vi "Start LabVIEW.vi"(8 "Error In":errorcluster, 11 "Install LV Data":T1={"SSH Session"=refnum, "Status Log"="", "Detailed Log"="", "Credentials"={"Hostname or IP"="192.168.7.2", "Username"="root", "Password"=""}, "Target Info"={"OS Version"="", "CPU"="", "Systemd Version"="", "Internet Access"=FALSE, "Device Type"="", "LV Installed Ver"="", "LV Available Ver"="", "LV Upgrade Available"=FALSE, "Hostname"="", "NIC Info"=[]}, "Reboot Required?"=FALSE}) -> (0 "Error Out":errorcluster, 1 "Log":string, 2 "LV Running?":bool, 3 "Install LV Data":T1={"SSH Session"=refnum, "Status Log"="", "Detailed Log"="", "Credentials"={"Hostname or IP"="192.168.7.2", "Username"="root", "Password"=""}, "Target Info"={"OS Version"="", "CPU"="", "Systemd Version"="", "Internet Access"=FALSE, "Device Type"="", "LV Installed Ver"="", "LV Available Ver"="", "LV Upgrade Available"=FALSE, "Hostname"="", "NIC Info"=[]}, "Reboot Required?"=FALSE})   [LabVIEW 2020, in "LMH-LINX.lvlib"]
uses:
  LMH-LINX.lvlib
  Install LV Data.ctl
  Target Info.ctl
  NIC Info.ctl
  NIC Mode.ctl
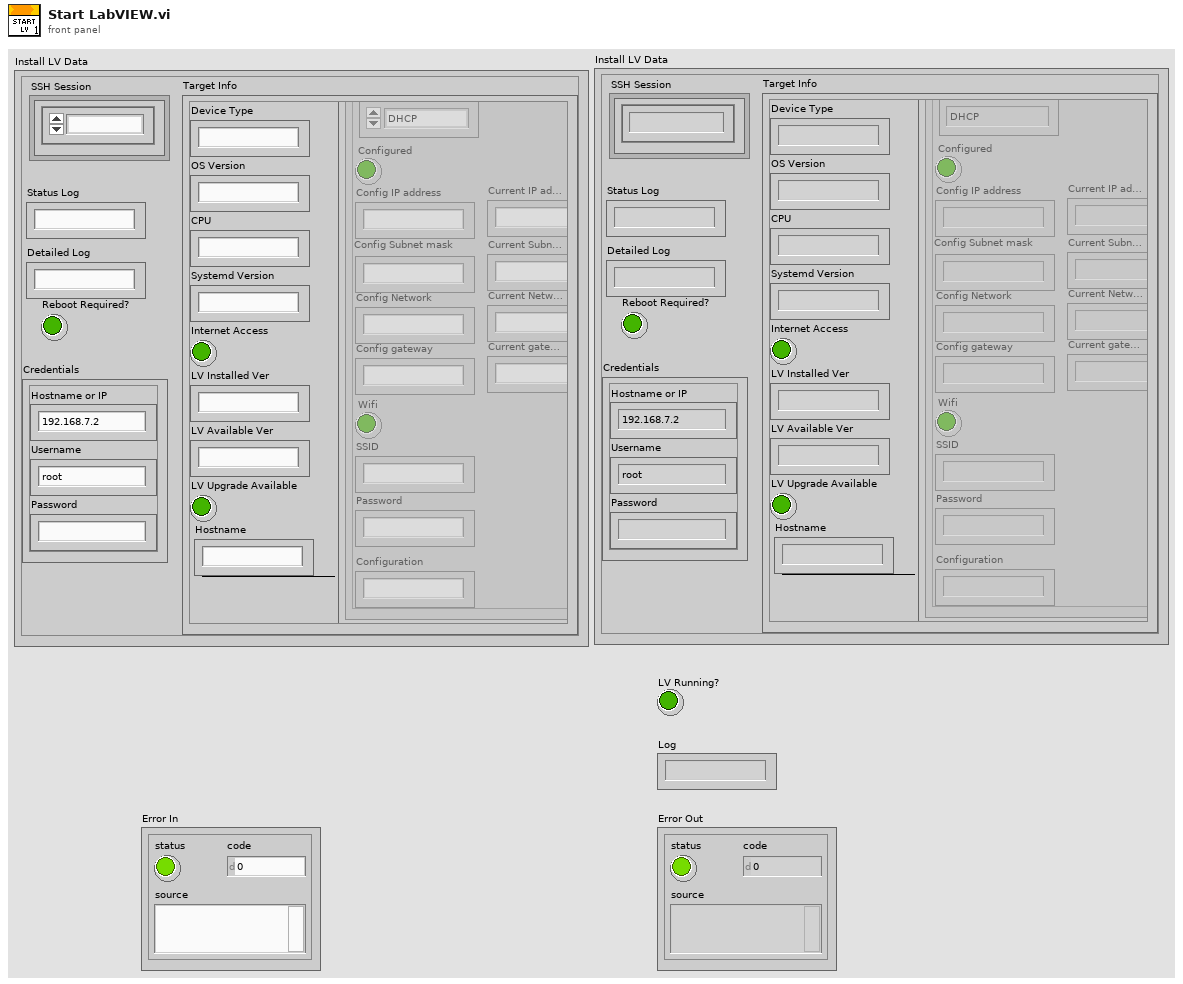
[diagram p1: front panel]
types:
  T1 = typedef "LMH-LINX.lvlib/Install LV Data.ctl" = cluster{"SSH Session":refnum<k1>, "Status Log":string, "Detailed Log":string, "Credentials":cluster{"Hostname or IP":string, "Username":string, "Password":string}, "Target Info":T2, "Reboot Required?":bool}
  T2 = typedef "LMH-LINX.lvlib/Target Info.ctl" = cluster{"OS Version":string, "CPU":string, "Systemd Version":string, "Internet Access":bool, "Device Type":string, "LV Installed Ver":string, "LV Available Ver":string, "LV Upgrade Available":bool, "Hostname":string, "NIC Info":T3[]}
  T3 = typedef "LMH-LINX.lvlib/NIC Info.ctl" = cluster{"Name":string, "NIC Mode":T4, "Configured":bool, "Config IP address":string, "Config Subnet mask":string, "Config Network":string, "Config gateway":string, "Wifi":bool, "SSID":string, "Password":string, "Configuration":string, "Current IP address":string, "Current Subnet mask":string, "Current gateway":string, "Current Network":string}
  T4 = typedef "LMH-LINX.lvlib/NIC Mode.ctl" = enum16{"DHCP", "Static", "Loopback"}
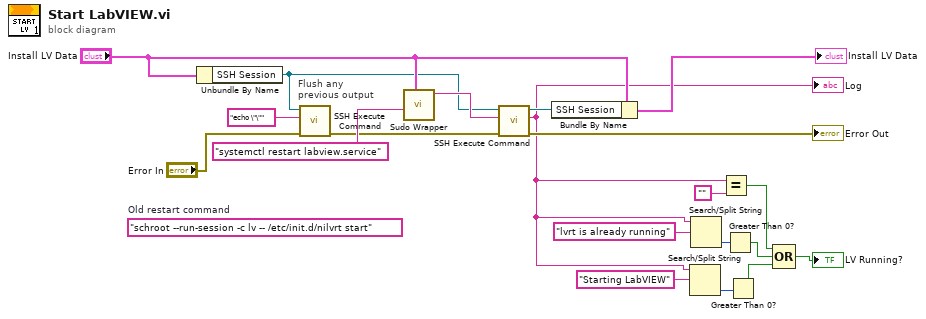
[diagram p0: block diagram]
diagram:
  (unwired) "schroot --run-session -c lv -- /etc/init.d/nilvrt start"  # Old restart command
  # "Flush any \nprevious output"
  n1 = Unbundle By Name("Install LV Data") -> ("SSH Session"=w4:refnum<k1>)
  n2 = call "SSH Execute Command.vi"("Error In"="Error In", "Command"="echo \"\"", "SSH Session"=w4) -> ("Error Out"=w1:errorcluster)  [unwired: 6 in, 2 out]
  n3 = call "Sudo Wrapper.vi"("Install LV Data"="Install LV Data", "comand string"="systemctl restart labview.service") -> ("combined command string"=w10:string)  [unwired: 9 in]
  n4 = call "SSH Execute Command.vi"("Error In"=w1, "Command"=w10, "SSH Session"=w4) -> ("Error Out"=→"Error Out":errorcluster, "Std Out"=w7:string, "SSH Session"=w12:refnum<k1>)  [unwired: 6 in]
  "Log" <- w7
  n5 = Bundle By Name(cluster="Install LV Data", "SSH Session"=w12) -> (→"Install LV Data":T1)
  n6 = Search/Split String(string=w7, search string/char (-)="Starting LabVIEW" ("regular expression")) -> (offset of match=w15:i32)  [unwired: 1 in, 2 out]
  n7 = Search/Split String(string=w7, search string/char (-)="lvrt is already running" ("regular expression")) -> (offset of match=w17:i32)  [unwired: 1 in, 2 out]
  n8 = Equal?(x=w7, y="") -> (x = y?=w5:bool)
  n9 = Greater Than 0?(x=w17) -> (x > 0?=w16:bool)
  n10 = Greater Than 0?(x=w15) -> (x > 0?=w14:bool)
  n11 = Compound Arithmetic op=OR(w5, w16, w14) -> (→"LV Running?":bool)
